vi "KE2260B Configure Voltage Slewrate.vi"(8 "error in (no error)":errorcluster, 9 "Slewrate Falling (0.01 V)":dbl=0.01 format="%.2g", 10 "Slewrate Rising (0.01 V)":dbl=0.01 format="%.2g", 11 "VISA resource name":refnum<visa-resource-name>) -> (0 "error out":errorcluster, 3 "VISA resource name out":refnum<visa-resource-name>)   [LabVIEW 2009, in "Keithley 2260B.lvlib"]
doc: "Configures the rising voltage slew rate and the falling voltage slew rate."
uses:
  <instrlib>/Keithley 2260B/Keithley 2260B.lvlib
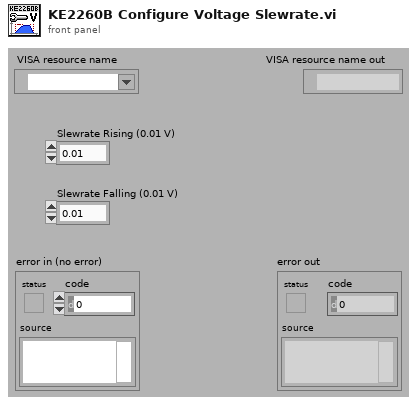
[diagram p1: front panel]
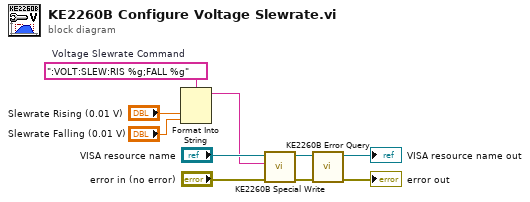
[diagram p0: block diagram]
diagram:
  w7 = ":VOLT:SLEW:RIS %g;FALL %g"  # Voltage Slewrate Command
  n1 = Format Into String(format string=w7, "Slewrate Rising (0.01 V)", "Slewrate Falling (0.01 V)") -> (resulting string=w2:string)  [unwired: 2 in, 1 out]
  n2 = call <instrlib>:"KE2260B Special Write.vi"("error in (no error)"="error in (no error)", "Write Buffer (\"\")"=w2, "VISA session"="VISA resource name") -> ("error out"=w6:errorcluster, "dup VISA session"=w5:refnum<visa-resource-name>)  [unwired: 6 in, 1 out]
  n3 = call <instrlib>:"KE2260B Error Query.vi"("error in (no error)"=w6, "VISA resource name"=w5) -> ("error out"=→"error out":errorcluster, "VISA resource name out"=→"VISA resource name out":refnum<visa-resource-name>)  [unwired: 6 in, 2 out]
